vi "Average_Table_Values.vi"(1 "Table values to average":dbl[][](array[numeric]) format="%.2f") -> (0 "Averaged Row":dbl[](array[numeric]) format="%.2f")   [LabVIEW 2010]
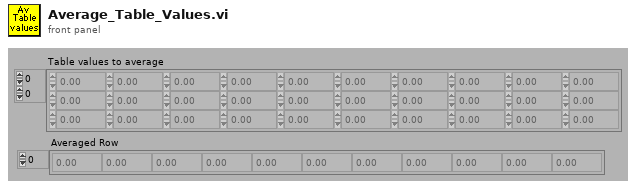
[diagram p1: front panel]
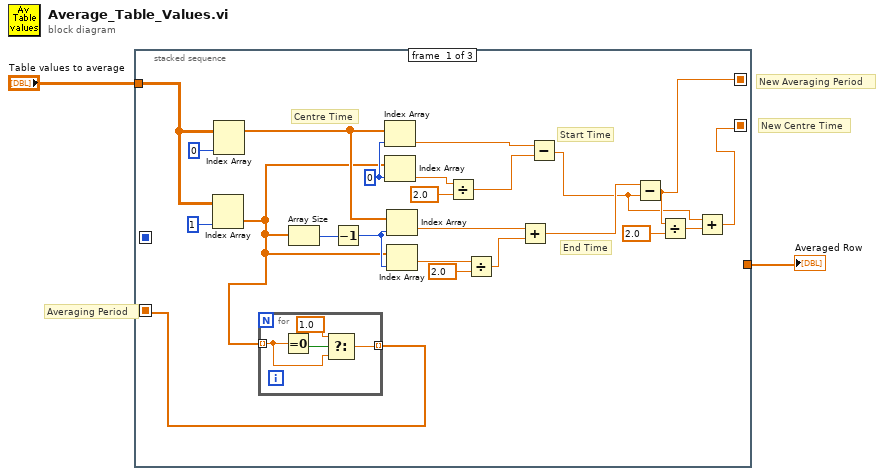
[diagram p0: block diagram]
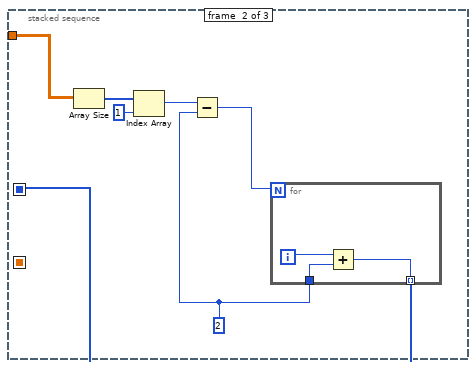
[diagram p2: hidden frame]
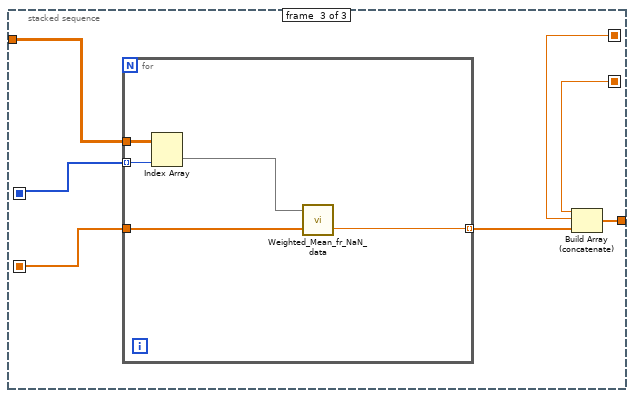
[diagram p3: hidden frame]
diagram:
  # "New Centre Time"
  # "New Averaging Period"
  # "Averaging Period"
  n1 = stacked-sequence {
    seq-local: [w3 _ _] -> [_ _ w44]
    seq-local: [w16 _ _] -> [_ _ w42]
    seq-local: [w12 _ _] -> [_ _ w43]
    seq-local: [_ w30 _] -> [_ _ w45]
    tunnel: "Table values to average" -> [w11 w36 w46]
    tunnel: [_ _ w40] -> w1
    frame #0 {
      w22 = 0 ("Index")
      # "End Time"
      # "Start Time"
      # "Centre Time"
      n2 = Index Array(array=w11, index (col)=1) -> (element=w4:dbl[])  [unwired: 1 in]
      n3 = Index Array(array=w11, index (col)=0) -> (element=w19:dbl[])  [unwired: 1 in]
      n4 = for {
        tunnel: w4 -> [w28] mode=indexing
        tunnel: [w26] -> w3 mode=indexing
        n5 = Equal To 0?(x=w28) -> (x = 0?=w29:bool)
        n6 = Select(t=1.0, s=w29, f=w28) -> (s? t:f=w26:dbl)
      }
      n7 = Array Size(array=w4) -> (size(s)=w23:i32)
      n8 = Decrement(x=w23) -> (x-1=w20:i32)
      n9 = Index Array(array=w19, index=w22) -> (element=w21:dbl)
      n10 = Index Array(array=w4, index=w22) -> (element=w9:dbl)
      n11 = Index Array(array=w19, index=w20) -> (element=w18:dbl)
      n12 = Index Array(array=w4, index=w20) -> (element=w6:dbl)
      n13 = Divide(x=w9, y=2.0) -> (x/y=w8:dbl)
      n14 = Divide(x=w6, y=2.0) -> (x/y=w5:dbl)
      n15 = Add(x=w18, y=w5) -> (x+y=w17:dbl)
      n16 = Subtract(x=w21, y=w8) -> (x-y=w14:dbl)
      n17 = Subtract(x=w17, y=w14) -> (x-y=w16:dbl)
      n18 = Divide(x=w16, y=2.0) -> (x/y=w13:dbl)
      n19 = Add(x=w14, y=w13) -> (x+y=w12:dbl)
    }
    frame #1 {
      w31 = 2 ("y")
      n20 = Array Size(array=w36) -> (size(s)=w35:i32[])
      n21 = Index Array(array=w35, index=1 ("Index")) -> (element=w33:i32)
      n22 = Subtract(x=w33, y=w31) -> (x-y=w32:i32)
      n23 = for {
        N: w32 -> [_]
        tunnel: w31 -> [w38]
        tunnel: [w37] -> w30 mode=indexing
        i -> [w39]
        n24 = Add(x=w39, y=w38) -> (x+y=w37:i32)
      }
    }
    frame #2 {
      n25 = for {
        tunnel: w46 -> [w51]
        tunnel: w45 -> [w50] mode=indexing
        tunnel: w44 -> [w48]
        tunnel: [w47] -> w41 mode=indexing
        n26 = Index Array(array=w51, index (col)=w50) -> (element=w49:dbl[])  [unwired: 1 in]
        n27 = call "Weighted_Mean_fr_NaN_data.vi"("Weighting"=w48, "Data"=w49) -> ("Mean value"=w47:dbl)
      }
      n28 = Build Array (concatenate)(w43, w42, w41) -> (w40:dbl[])
    }
  }
  "Averaged Row" <- w1
